vi "Get Active Options.vi"(11 "Car Wash Console in":refnum<class "Car Wash Console.lvclass">) -> (3 "Car Wash Console out":refnum<class "Car Wash Console.lvclass">, 4 "Options":string[](array[string]))   [LabVIEW 2016, in "CLD Exam - Car Wash.lvlib" / "Car Wash Console.lvclass"]
uses:
  Car Wash Console.lvclass
  Car Wash Console.lvclass/Car Wash Console.ctl
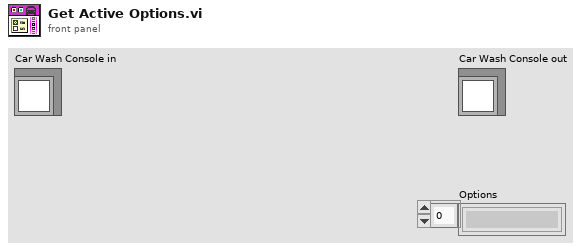
[diagram p1: front panel]
types:
  T1 = cluster{"Alpha":refnum<vi>, "Air Dry":refnum<vi>, "Tire Shine Foam":refnum<vi>, "Spot Free Rinse":refnum<vi>, "Low Pressure Wash":refnum<vi>, "High Pressure Wash":refnum<vi>, "Pre-Soak":refnum<vi>, "Bug Remover":refnum<vi>, "Under Body Wash":refnum<vi>}
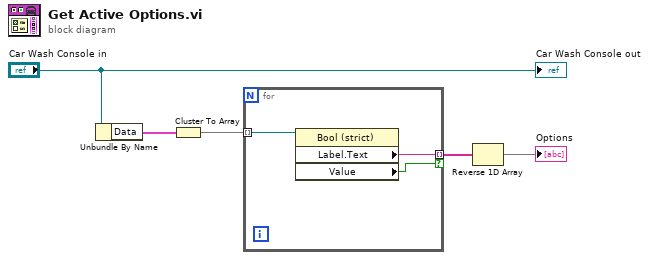
[diagram p0: block diagram]
diagram:
  n1 = Unbundle By Name("Car Wash Console in") -> ("Data"=w4:T1)
  n2 = Cluster To Array(cluster=w4) -> (array=w3:refnum<vi>[])
  n3 = for {
    tunnel: w3 -> [w8] mode=indexing
    tunnel: [w7] -> w2 mode=indexing if=w6
    n4 = property class="Bool (strict)"(reference=w8) -> ("Label.Text"=w7:string, "Value"=w6:bool)  [unwired: 1 in, 2 out]
  }
  n5 = Reverse 1D Array(array=w2) -> (reversed array=→"Options":string[])
  "Car Wash Console out" <- "Car Wash Console in"
